vi "Read_supply_with_boardhandle.vi"(8 "error in (no error)":errorcluster, 11 "BoardHandle":T1) -> (0 "error out":errorcluster, 1 "IMon values (uA)":dbl[](array[numeric]) format="%.2f", 2 "VMon values (V)":dbl[](array[numeric]) format="%.1f", 3 "BoardHandle out":T1)   [LabVIEW 2018]
uses:
  <instrlib>/CAEN PSM/CAEN PSM.lvlib
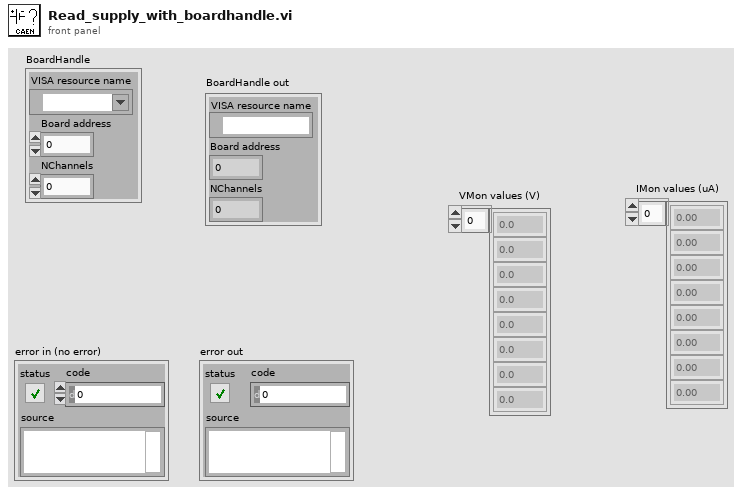
[diagram p1: front panel]
types:
  T1 = cluster{"VISA resource name":refnum<visa-resource-name>, "Board address":u8, "NChannels":u8}
  T2 = typedef "CAEN PSM.lvlib/BoardHandle.ctl" = cluster{"VISA resource name":refnum<visa-resource-name>, "Board address":u8, "NChannels":u8}
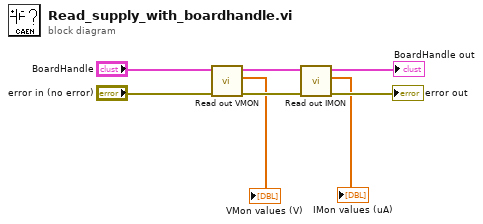
[diagram p0: block diagram]
diagram:
  n1 = call <instrlib>:"Read out VMON.vi"("error in (no error)"="error in (no error)", "BoardHandle"="BoardHandle") -> ("error out"=w5:errorcluster, "VMon values (V)"=→"VMon values (V)":dbl[], "BoardHandle out"=w4:T2)  [unwired: 7 in]
  n2 = call <instrlib>:"Read out IMON.vi"("error in (no error)"=w5, "BoardHandle"=w4) -> ("error out"=→"error out":errorcluster, "IMon values (uA)"=→"IMon values (uA)":dbl[], "BoardHandle out"=→"BoardHandle out":T2)  [unwired: 6 in, 1 out]
